vi "Convert LabVIEW Image Data To IMAQ.vi"(8 "error in":errorcluster, 10 "Image Data":T1, 11 "Image In":T2) -> (0 "error out":errorcluster, 3 "Image Out":T2)   [LabVIEW 2024, in "IMAQ Helpers.lvlib"]
doc: "This VI converts a LabVIEW Image into an IMAQ image."
uses:
  IMAQ Helpers.lvlib
  <vilib>/vision/Image Controls.llb/IMAQ Image.ctl
  <vilib>/picture/picture.llb/imagedata.ctl
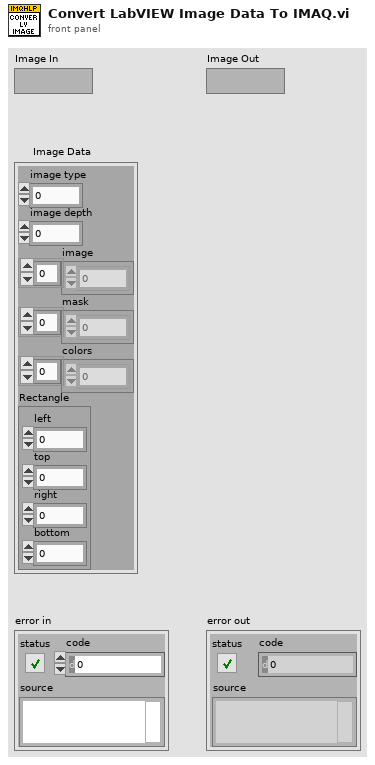
[diagram p1: front panel]
types:
  T1 = typedef "imagedata.ctl" = cluster{"image type":i32, "image depth":i32, "image":u8[], "mask":u8[], "colors":u32[], "Rectangle":cluster{"left":i16, "top":i16, "right":i16, "bottom":i16}}
  T2 = typedef "IMAQ Image.ctl" = refnum<image>
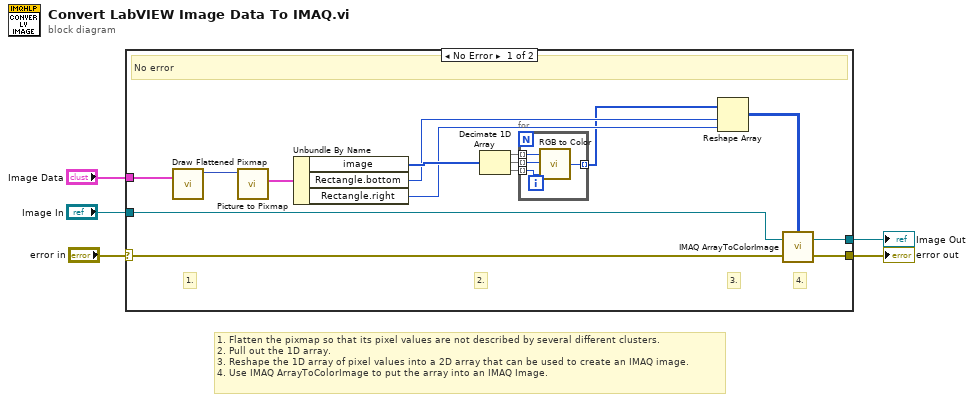
[diagram p0: block diagram]
diagram:
  # "1. Flatten the pixmap so that its pixel values are not described by several different clusters.\n2. Pull out the 1D array.\n3. Reshape the 1D array of pixel values into a 2D array that can be used to create an IMAQ image.\n4. Use IMAQ ArrayToColorImage to put the array into an IMAQ Image."
  n1 = case shown="No Error" "error in" {
    selector: "error in" -> [w7 w26]
    tunnel: [w14 w25] -> w5
    tunnel: [w13 w26] -> w4
    tunnel: "Image In" -> [w12 w25]
    tunnel: "Image Data" -> [w6 _]
    frame No Error {
      # "4."
      # "3."
      # "2."
      # "1."
      # "No error"
      n2 = call <vilib>:"Draw Flattened Pixmap.vi"("image data"=w6) -> ("new picture"=w20:picture)  [unwired: 8 in]
      n3 = call <vilib>:"Picture to Pixmap.vi"("picture"=w20) -> ("image data"=w19:T1)  [unwired: 9 in, 1 out]
      n4 = Unbundle By Name(w19) -> ("image"=w18:u8[], "Rectangle.bottom"=w17:i16, "Rectangle.right"=w16:i16)
      n5 = Decimate 1D Array(w18) -> (w11:u8[], w10:u8[], w9:u8[])
      n6 = for {
        tunnel: w11 -> [w24] mode=indexing
        tunnel: w10 -> [w23] mode=indexing
        tunnel: w9 -> [w22] mode=indexing
        tunnel: [w21] -> w8 mode=indexing
        n7 = call <vilib>:"RGB to Color.vi"("B"=w22, "G"=w23, "R"=w24) -> ("Color"=w21:u32)
      }
      n8 = Reshape Array(w8, w17, w16) -> (w15:u32[][])
      n9 = call "IMAQ ArrayToColorImage"("Image Pixels (U32)"=w15, "Image"=w12, "error in (no error)"=w7) -> ("Image Out"=w14:T2, "error out"=w13:errorcluster)  [unwired: 2 in]
    }
    frame Error {
      # "Error"
    }
  }
  "Image Out" <- w5
  "error out" <- w4
